vi "Check Bitfile Register Names.vi"(8 "error in (no error)":errorcluster, 10 "RegisterMap in":T1[](array[typedef]) {"Address" format="%.0x"}) -> (0 "error out":errorcluster, 2 "RegisterMap out":T1[](array[typedef]) {"Address" format="%.0x"})   [LabVIEW 2023, in "FPGA Addon System Explorer.lvlib"]
uses:
  FPGA Addon System Explorer.lvlib
  <userlib>/_OpenG.lib/array/array.llb/openg_array.lvlib
  <userlib>/_OpenG.lib/array/array.llb/Remove Duplicates from 1D Array (String)__ogtk.vi
  <vilib>/rvi/Bitfile/nirviTypdefDescription.ctl
  <vilib>/rvi/Bitfile/nirviMechanicalAction.ctl
  <vilib>/rvi/Bitfile/nirviClusterElementControl.ctl
  <vilib>/rvi/Bitfile/nirviSubControlStructure.ctl
  <vilib>/rvi/Bitfile/nirviControlStructure.ctl
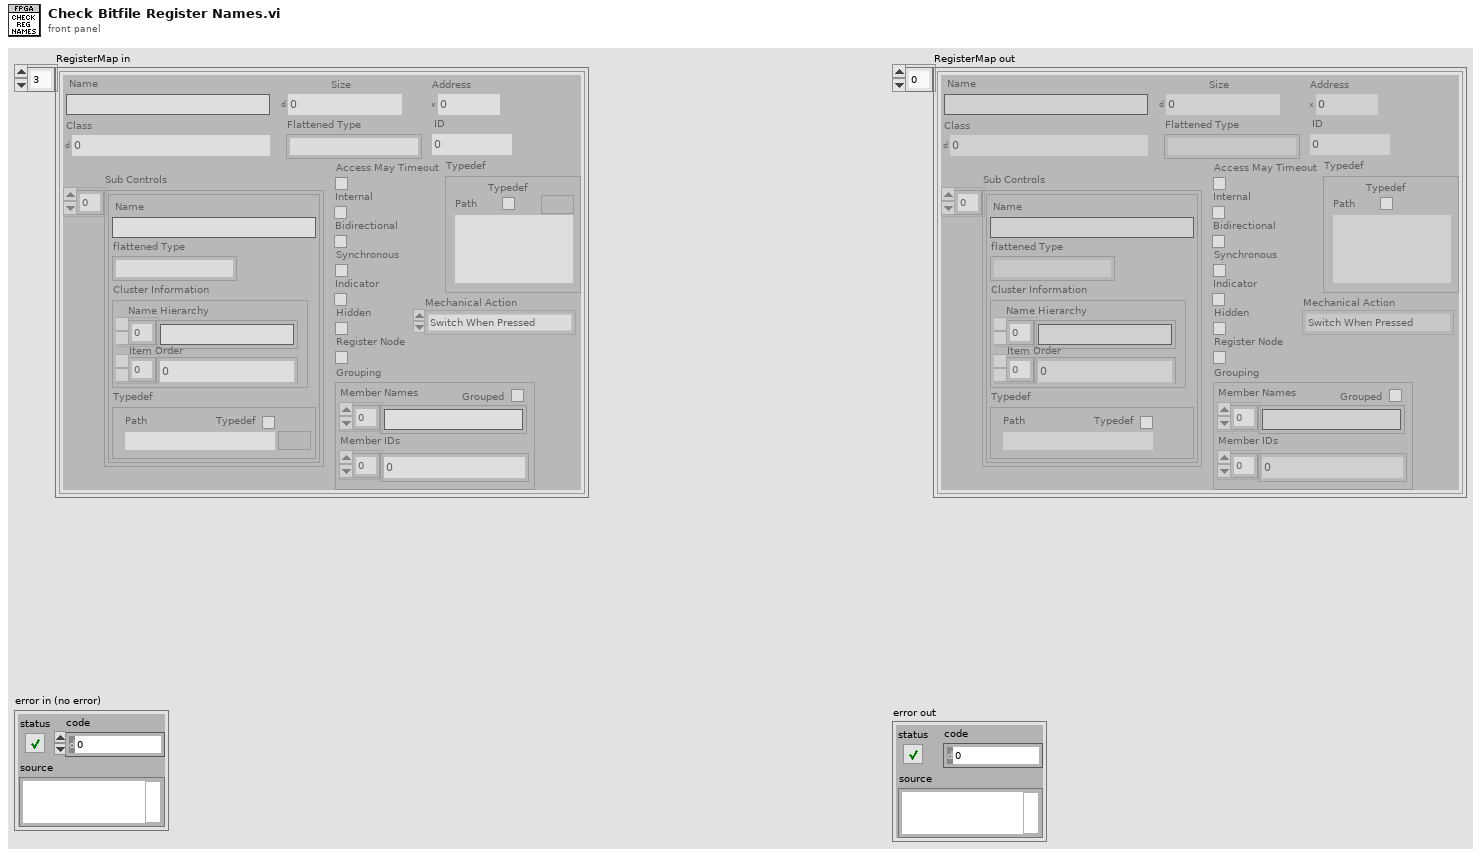
[diagram p1: front panel]
types:
  T1 = typedef "nirviControlStructure.ctl" = cluster{"Name":string, "Hidden":bool, "Indicator":bool, "Flattened Type":string, "Grouping":cluster{"Grouped":bool, "Member Names":string[], "Member IDs":u32[]}, "Address":u32, "Size":u32, "Class":u32, "Internal":bool, "Typedef":T2, "ID":u32, "Bidirectional":bool, "Synchronous":bool, "Mechanical Action":T3, "Sub Controls":T4[], "Access May Timeout":bool, "Register Node":bool}
  T2 = typedef "nirviTypdefDescription.ctl" = cluster{"Typedef":bool, "Path":path}
  T3 = typedef "nirviMechanicalAction.ctl" = enum8{"Switch When Pressed", "Switch When Released", "Switch Until Released", "Latch When Pressed", "Latch When Released", "Latch Until Released"}
  T4 = typedef "nirviSubControlStructure.ctl" = cluster{"Name":string, "flattened Type":string, "Cluster Information":T5, "Typedef":T2}
  T5 = typedef "nirviClusterElementControl.ctl" = cluster{"Name Hierarchy":string[], "Item Order":u32[]}
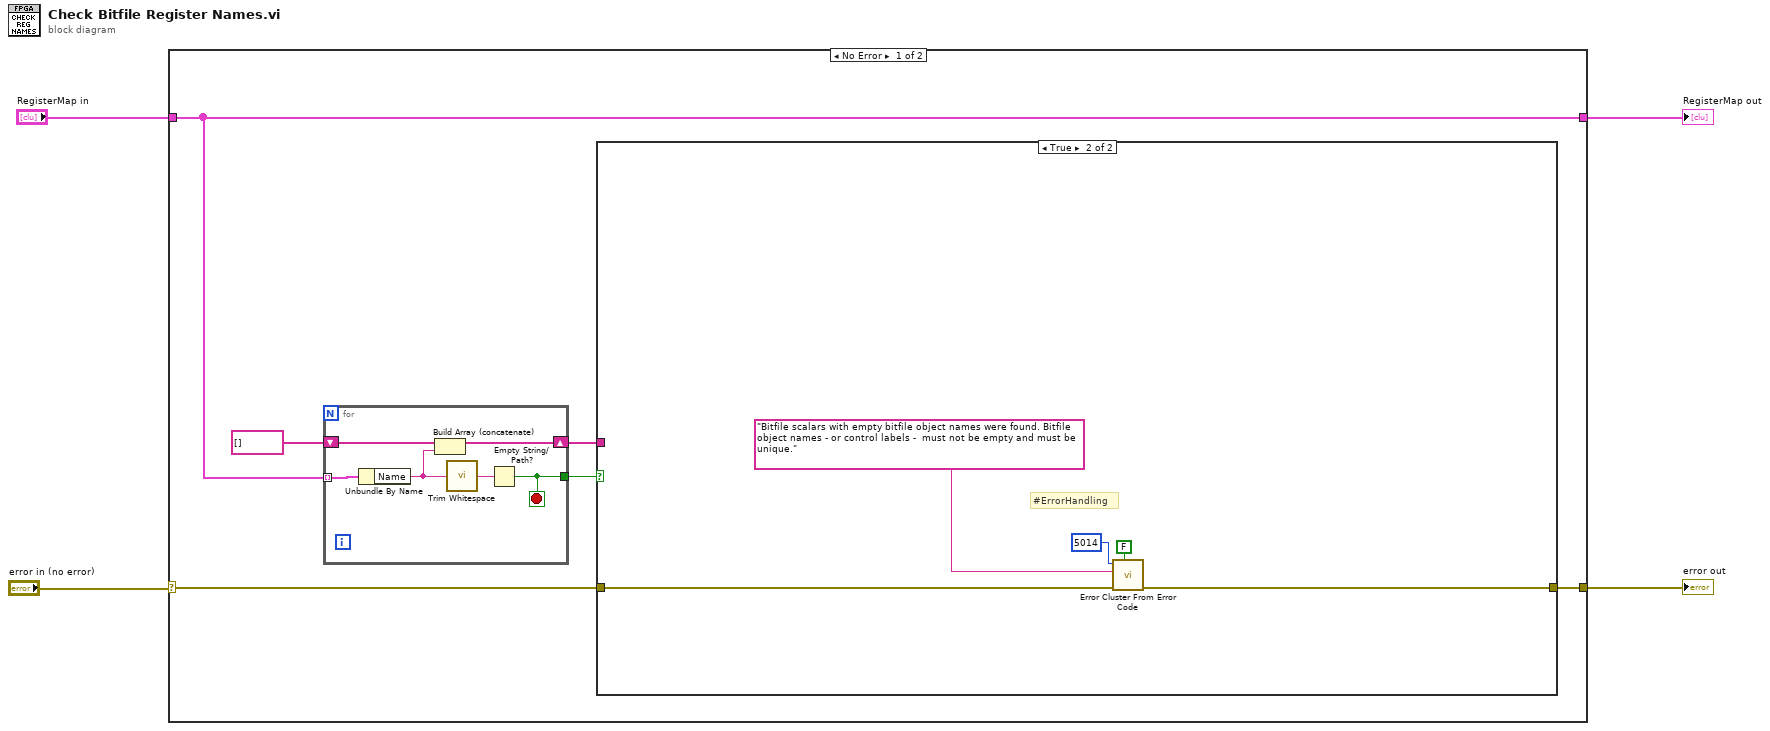
[diagram p0: block diagram]
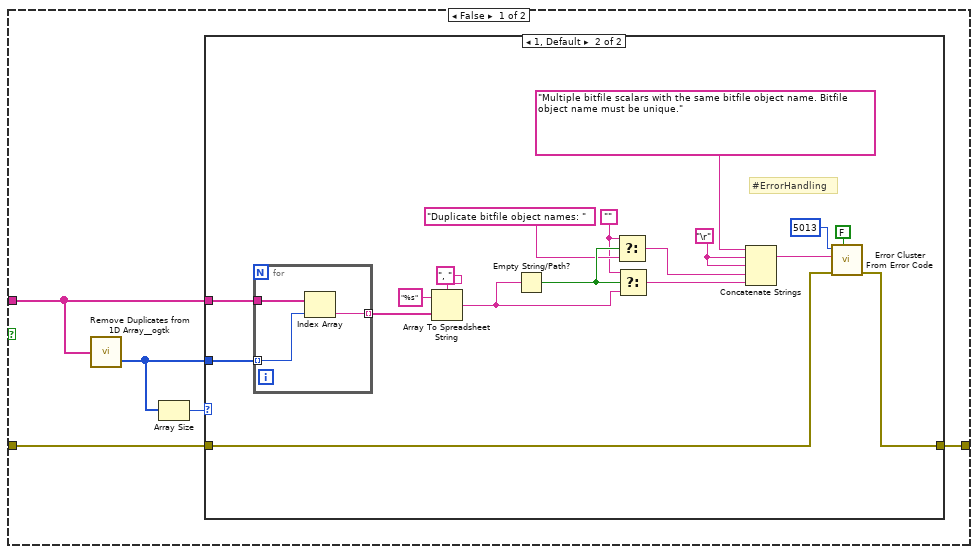
[diagram p2: hidden frame]
diagram:
  n1 = case shown="No Error" "error in (no error)" {
    selector: "error in (no error)" -> [w7 w50]
    tunnel: "RegisterMap in" -> [w9 w49]
    tunnel: [w6 w50] -> w2
    tunnel: [w9 w49] -> w1
    frame No Error {
      n2 = for {
        tunnel: w9 -> [w48] mode=indexing
        shift-right: [w46] -> w8
        shift-left: string[] [] ("appended array") -> [w47]
        tunnel: [w43] -> w5
        stop <- w43 stop-if-true
        n3 = Unbundle By Name(w48) -> ("Name"=w45:string)
        n4 = Build Array (concatenate)(w47, w45) -> (w46:string[])
        n5 = call <vilib>:"Trim Whitespace.vi"("string"=w45) -> ("trimmed string"=w44:string)  [unwired: 1 in]
        n6 = Empty String/Path?(string/path=w44) -> (empty?=w43:bool)
      }
      n7 = case shown="True" w5 {
        tunnel: w8 -> [w14 _]
        tunnel: w7 -> [w12 w39]
        tunnel: [w11 w38] -> w6
        frame False {
          n8 = call-poly <userlib>:"Remove Duplicates from 1D Array__ogtk.vi"("Input Array"=w14) -> ("indices of removed elements"=w13:i32[])  [unwired: 1 out]
          n9 = Array Size(array=w13) -> (size(s)=w15:i32)
          n10 = case shown="1, Default" w15 {
            tunnel: w14 -> [_ w33]
            tunnel: w13 -> [_ w34]
            tunnel: w12 -> [w16 w18]
            tunnel: [w16 w17] -> w11
            frame 0 {
            }
            frame 1, Default {
              w24 = "\r"
              w26 = ""
              # "#ErrorHandling"
              n11 = for {
                tunnel: w34 -> [w36] mode=indexing
                tunnel: w33 -> [w37]
                tunnel: [w35] -> w19 mode=indexing
                n12 = Index Array(array=w37, index=w36) -> (element=w35:string)
              }
              n13 = Array To Spreadsheet String(delimiter (Tab)=", ", array=w19, 3:"%s" ("format string")) -> (spreadsheet string=w30:string)
              n14 = Empty String/Path?(string/path=w30) -> (empty?=w29:bool)
              n15 = Select(t=w26, s=w29, f="Duplicate bitfile object names: " ("string")) -> (s? t:f=w31:string)
              n16 = Select(t=w26, s=w29, f=w30) -> (s? t:f=w32:string)
              n17 = Concatenate Strings("Multiple bitfile scalars with the same bitfile object name. Bitfile object name must be unique." ("error message (\"\")"), w24, w24, w31, w32) -> (w28:string)
              n18 = call <vilib>:"Error Cluster From Error Code.vi"("show call chain? (False)"=FALSE, "error in (no error)"=w18, "error message (\"\")"=w28, "error code (0)"=5013) -> ("error out"=w17:errorcluster)  [unwired: 5 in]
            }
          }
        }
        frame True {
          # "#ErrorHandling"
          n19 = call <vilib>:"Error Cluster From Error Code.vi"("show call chain? (False)"=FALSE, "error in (no error)"=w39, "error message (\"\")"="Bitfile scalars with empty bitfile object names were found. Bitfile object names - or control labels -  must not be empty and must be unique." ("error message (\"\")"), "error code (0)"=5014) -> ("error out"=w38:errorcluster)  [unwired: 5 in]
        }
      }
    }
    frame Error {
    }
  }
  "error out" <- w2
  "RegisterMap out" <- w1
